vi "Update Witness Name.vi"(8 "error in":errorcluster, 10 "Witness_Name":string, 11 "Report Generator in":refnum<class "Report Generator.lvclass">) -> (0 "error out":errorcluster, 3 "Report Generator out":refnum<class "Report Generator.lvclass">)   [LabVIEW 2019, in "Report Generator.lvlib" / "Report Generator.lvclass"]
uses:
  Library/Report Generator.lvclass
  C:/Users/Public/Documents/Development/builds/Engine/Engine.lvlibp/Project/Engine.lvclass
  Library/Report Generator.lvclass/Report Generator.ctl
  builds/Engine/Engine.lvlibp/Accessors/Read Self Q.vi
  builds/Engine/Actor Framework.lvlibp/1abvi3w/vi.lib/ActorFramework/Message Enqueuer/Enqueue.vi
  builds/Engine/Actor Framework.lvlibp/1abvi3w/vi.lib/ActorFramework/Message Enqueuer/Message Enqueuer.lvclass
  Report Generator Messages/Prepare Test Naming Msg/Prepare Test Naming Msg.lvclass
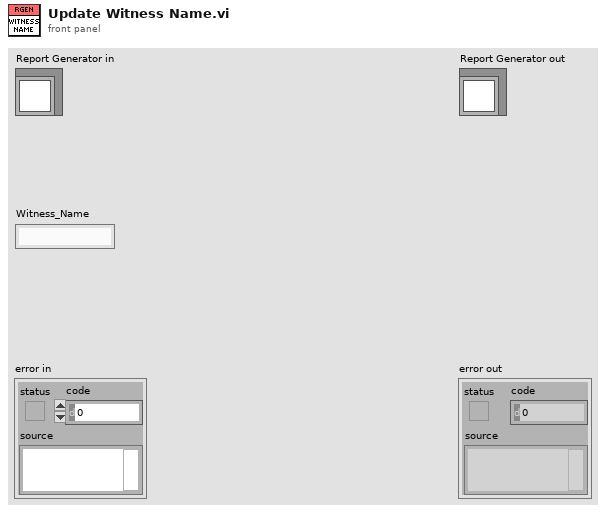
[diagram p1: front panel]
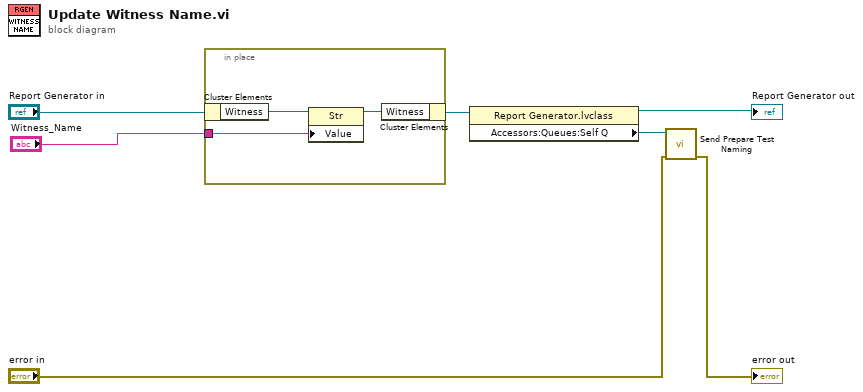
[diagram p0: block diagram]
diagram:
  n1 = in-place {
    in-place-border: "Witness_Name" -> [w9]
    n2 = in-place-cluster #1("Report Generator in") -> ("Witness"=w10:refnum<vi>)
    n3 = property class="Str"(reference=w10, "Value"=w9) -> (reference out=w8:refnum<vi>)  [unwired: 1 in, 1 out]
    n4 = in-place-cluster #1("Witness"=w8) -> (w4:refnum<class "Report Generator.lvclass">)
  }
  n5 = property class="Report Generator.lvclass"(reference=w4) -> (reference out=→"Report Generator out":refnum<class "Report Generator.lvclass">, "Accessors:Queues:Self Q"=w5:refnum<class "Message Enqueuer.lvclass">)  [unwired: 1 in, 1 out]
  n6 = call "Send Prepare Test Naming.vi"("error in (no error)"="error in", "Message Enqueuer"=w5) -> ("error out"=→"error out":errorcluster)  [unwired: 8 in, 1 out]
